vi "Header_CF.vi"(1 "Cluster":T1={"Multiply Data?"=TRUE, "Configuration"=enum."Preamp", "Preamp Sensitivity"=enum."1nA/V", "Step Time (sec)"=0.5, "Output 1"=0.0, "Output 2"=0.0, "Preamp Bias (mv)"=0, "Preamp Bias on?"=FALSE, "Wavelength:"=1010.0, "Use Current offset"=TRUE, "Current offset"=0.0, "Y scale 1"="", "x scale"=""} {"Wavelength:" min=0.0 max=2000.0 step=0.1 format="%.1f"; "Output 2" step=0.05; "Output 1" step=0.01; "Step Time (sec)" min=0.001 max=300.0 step=0.001 format="%.3f"}, 2 "String in":string) -> (0 "String out":string)   [LabVIEW 2013]
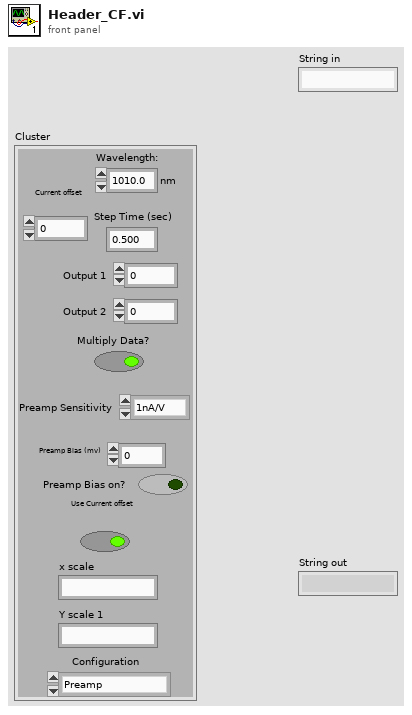
[diagram p1: front panel]
types:
  T1 = cluster{"Multiply Data?":bool, "Configuration":enum16{"Preamp to Lockin", "Preamp", "Lockin current", "Lockin Voltage", ""}, "Preamp Sensitivity":enum16{"1pA/V", "2pA/V", "5pA/V", "10pA/V", "20pA/V", "50pA/V", "100pA/V", "200pA/V", "500pA/V", "1nA/V", "2nA/V", "5nA/V", "10nA/V", "20nA/V", "50nA/V", "100nA/V", "200nA/V", "500nA/V", "1uA/V", "2uA/V", "5uA/V", "10uA/V", "20uA/V", "50uA/V", "100uA/V", "200uA/V", "500uA/V", "1mA/V"}, "Step Time (sec)":dbl, "Output 1":dbl, "Output 2":dbl, "Preamp Bias (mv)":i32, "Preamp Bias on?":bool, "Wavelength:":dbl, "Use Current offset":bool, "Current offset":dbl, "Y scale 1":string, "x scale":string}
  T2 = enum16{"Preamp to Lockin", "Preamp", "Lockin current", "Lockin Voltage", ""}
  T3 = enum16{"1pA/V", "2pA/V", "5pA/V", "10pA/V", "20pA/V", "50pA/V", "100pA/V", "200pA/V", "500pA/V", "1nA/V", "2nA/V", "5nA/V", "10nA/V", "20nA/V", "50nA/V", "100nA/V", "200nA/V", "500nA/V", "1uA/V", "2uA/V", "5uA/V", "10uA/V", "20uA/V", "50uA/V", "100uA/V", "200uA/V", "500uA/V", "1mA/V"}
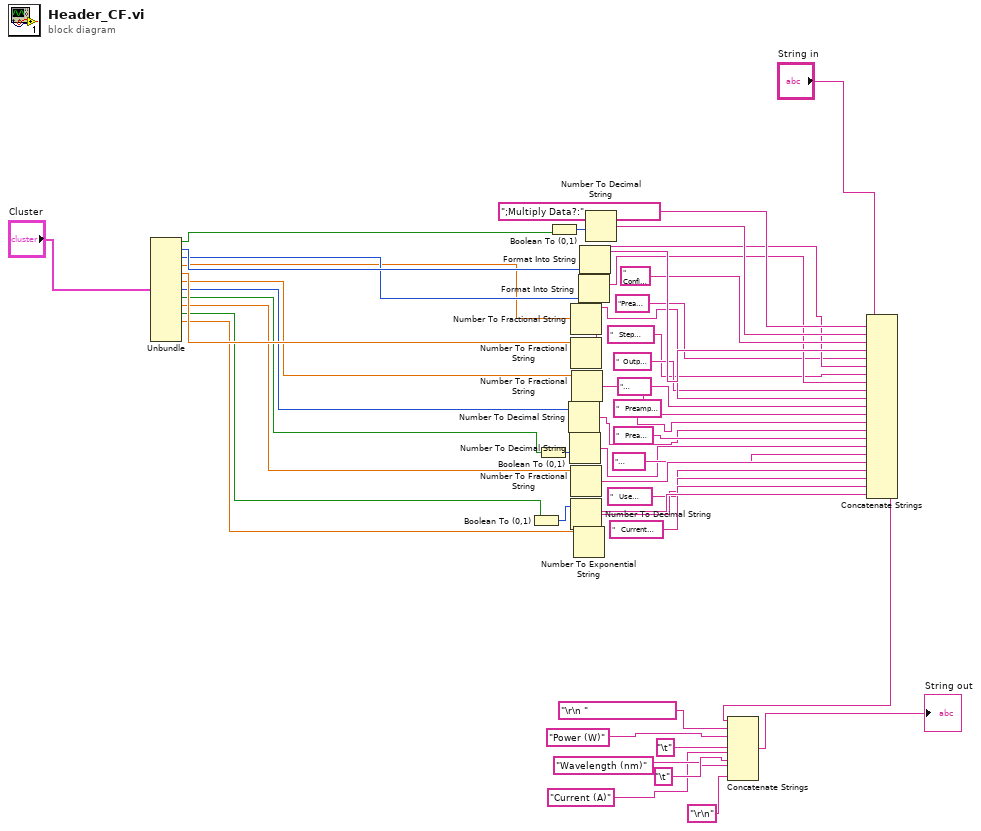
[diagram p0: block diagram]
diagram:
  n1 = Unbundle("Cluster") -> ("Multiply Data?"=w15:bool, "Configuration"=w14:T2, "Preamp Sensitivity"=w13:T3, "Step Time (sec)"=w12:dbl, "Output 1"=w11:dbl, "Output 2"=w10:dbl, "Preamp Bias (mv)"=w9:i32, "Preamp Bias on?"=w8:bool, "Wavelength:"=w7:dbl, "Use Current offset"=w6:bool, "Current offset"=w5:dbl)  [unwired: 2 out]
  n2 = Boolean To (0,1)(Boolean=w6) -> (0, 1=w43:i16)
  n3 = Boolean To (0,1)(Boolean=w8) -> (0, 1=w19:i16)
  n4 = Boolean To (0,1)(Boolean=w15) -> (0, 1=w34:i16)
  n5 = Number To Decimal String(number=w9) -> (decimal integer string=w27:string)  [unwired: 1 in]
  n6 = Number To Decimal String(number=w19) -> (decimal integer string=w29:string)  [unwired: 1 in]
  n7 = Number To Fractional String(number=w12) -> (F-format string=w22:string)  [unwired: 3 in]
  n8 = Number To Fractional String(number=w11) -> (F-format string=w24:string)  [unwired: 3 in]
  n9 = Number To Fractional String(number=w7) -> (F-format string=w37:string)  [unwired: 3 in]
  n10 = Number To Decimal String(number=w43) -> (decimal integer string=w45:string)  [unwired: 1 in]
  n11 = Number To Fractional String(number=w10) -> (F-format string=w42:string)  [unwired: 3 in]
  n12 = Number To Exponential String(number=w5) -> (E-format string=w47:string)  [unwired: 3 in]
  n13 = Format Into String(w13) -> (resulting string=w30:string)  [unwired: 3 in, 1 out]
  n14 = Format Into String(w14) -> (resulting string=w32:string)  [unwired: 3 in, 1 out]
  n15 = Number To Decimal String(number=w34) -> (decimal integer string=w35:string)  [unwired: 1 in]
  n16 = Concatenate Strings("String in", ";Multiply Data?:" ("string"), w35, "  Configuration:" ("string"), w32, "Preamp Sensitivity:" ("string"), w30, "   Step Time:" ("string"), w22, "  Output 1 :" ("string"), w24, "   Output 2:" ("string"), w42, "   Preamp Bias:" ("string"), w27, "   Preamp Bias on: " ("string"), w29, "   Wavelength: " ("string"), w37, "   Use Current offset: " ("string"), w45, "   Current offset: " ("string"), w47) -> (w38:string)
  n17 = Concatenate Strings(w38, "\r\n " ("string"), "Power (W)", "\t" ("string"), "Current (A)", "\t" ("string"), "Wavelength (nm)", "\r\n" ("string")) -> (→"String out":string)
